vi "Process-error.vi"(8 "error in (no error)":errorcluster, 11 "Data ref. in":refnum<data-value>) -> (0 "error out":errorcluster, 3 "Data ref.":refnum<data-value>)   [LabVIEW 2013, in "CameraVision.lvlib" / "CV-Main.lvclass"]
uses:
  CV-Main.lvclass
  CV-Main.lvclass/CV-Main.ctl
  Errors/CV-Errors.lvclass/CV-Errors.ctl
  Read Errors.vi
  Errors/Read Language.vi
  Errors/Read Display error dialog.vi
  Errors/CV-Errors.lvclass
  Client/Sources/CV-Client.lvclass
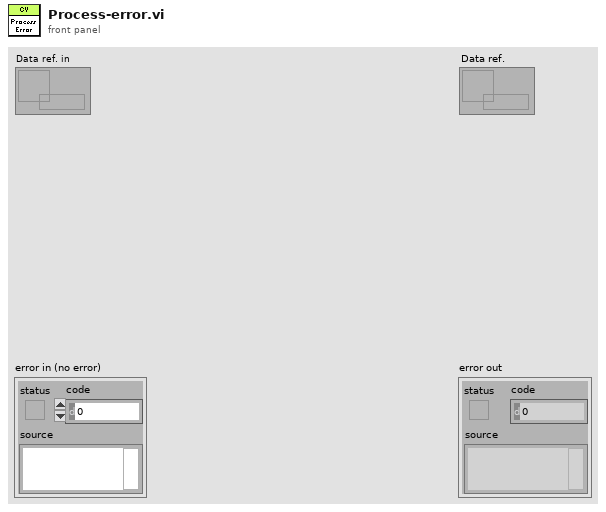
[diagram p1: front panel]
types:
  T1 = typedef "CameraVision.lvlib/CV-Errors.lvclass/Object-reference.ctl" = refnum<data-value>
  T2 = typedef "CameraVision.lvlib/CV-Errors.lvclass/Languages.ctl" = enum16{"English"}
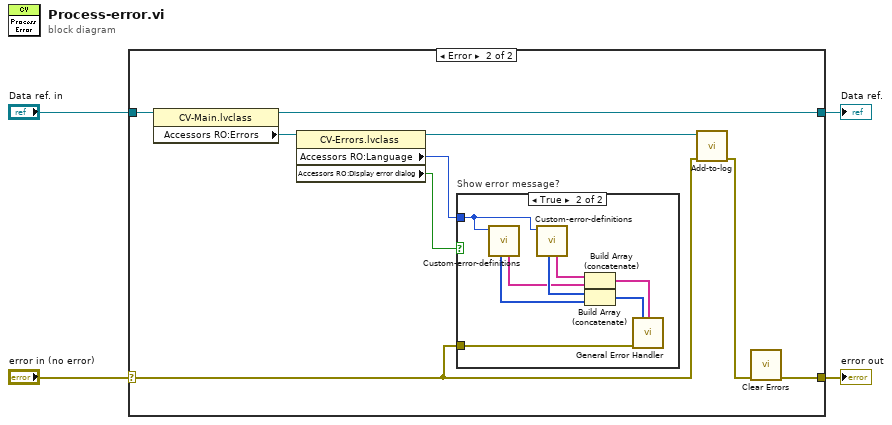
[diagram p0: block diagram]
diagram:
  n1 = case shown="Error" "error in (no error)" {
    selector: "error in (no error)" -> [w5 w7]
    tunnel: [w5 w13] -> w3
    tunnel: [w6 w10] -> w1
    tunnel: "Data ref. in" -> [w6 w14]
    frame No Error {
    }
    frame Error {
      n2 = property class="CV-Main.lvclass"(reference=w14) -> (reference out=w10:refnum<data-value>, "Accessors RO:Errors"=w12:T1)  [unwired: 1 in, 1 out]
      n3 = property class="CV-Errors.lvclass"(reference=w12) -> (reference out=w11:T1, "Accessors RO:Language"=w9:T2, "Accessors RO:Display error dialog"=w8:bool)  [unwired: 1 in, 1 out]
      n4 = case "Show error message?" shown="True" w8 {
        tunnel: w7 -> [_ w23]
        tunnel: w9 -> [_ w22]
        frame False {
        }
        frame True {
          n5 = call "Custom-error-definitions.vi"("Language"=w22) -> ("Descriptions"=w19:string[], "Error codes"=w18:i32[])  [unwired: 8 in, 1 out]
          n6 = call "Custom-error-definitions.vi"("Language"=w22) -> ("Descriptions"=w21:string[], "Error codes"=w20:i32[])  [unwired: 8 in, 1 out]
          n7 = Build Array (concatenate)(w21, w19) -> (w17:string[])
          n8 = Build Array (concatenate)(w20, w18) -> (w16:i32[])
          n9 = call <vilib>:"General Error Handler.vi"("[user-defined codes]"=w16, "[user-defined descriptions]"=w17, "error in (no error)"=w23) -> ()  [unwired: 8 in, 5 out]
        }
      }
      n10 = call "Add-to-log.vi"("error in (no error)"=w7, "Errors in"=w11) -> ("error out"=w15:errorcluster)  [unwired: 8 in, 1 out]
      n11 = call <vilib>:"Clear Errors.vi"("error in (no error)"=w15) -> ("error out"=w13:errorcluster)  [unwired: 6 in]
    }
  }
  "error out" <- w3
  "Data ref." <- w1
